vi "Auto Shooter Loop.vi"(4 "Right Shooter RPM":dbl, 6 "Left Shooter RPM":dbl, 10 "Vision Packet":T1, 11 "Shooter Presets":T2) -> ()   [LabVIEW 2016]
uses:
  Robot Global Data.vi
  Common Code/Auto Shoot Commands.ctl
  Common Code/Shooter Presets.ctl
  Common Code/Vision Packet.ctl
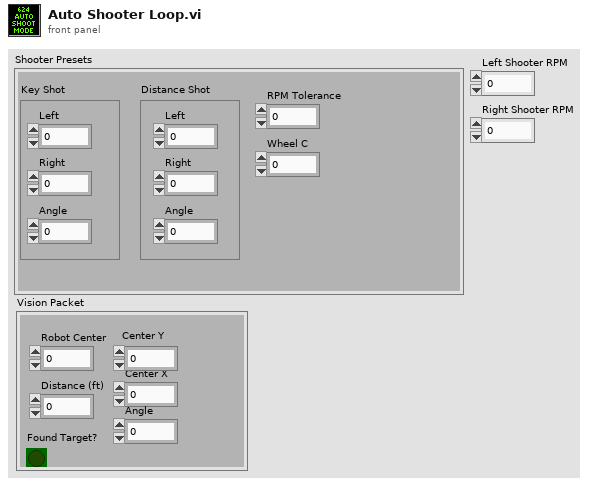
[diagram p1: front panel]
types:
  T1 = typedef "Vision Packet.ctl" = cluster{"Robot Center ":dbl, "Distance (ft)":dbl, "Center X":dbl, "Center Y":dbl, "Angle":dbl, "Found Target?":bool}
  T2 = typedef "Shooter Presets.ctl" = cluster{"Key Shot":cluster{"Left ":dbl, "Right":dbl, "Angle":dbl}, "Distance Shot":cluster{"Left":dbl, "Right":dbl, "Angle":dbl}, "RPM Tolerance":dbl, "Wheel C":dbl}
  T3 = typedef "Auto Shoot Commands.ctl" = enum16{"Idle", "Warmup", "Shoot"}
  T4 = typedef "Shooter Command Cluster.ctl" = cluster{"Y Power":dbl, "Modes":T5, "Shot Types":T6, "Auto Commands":T3}
  T5 = typedef "Shooter Modes.ctl" = enum16{"Manual", "Auto"}
  T6 = typedef "Shot Types.ctl" = enum16{"Key", "Distance"}
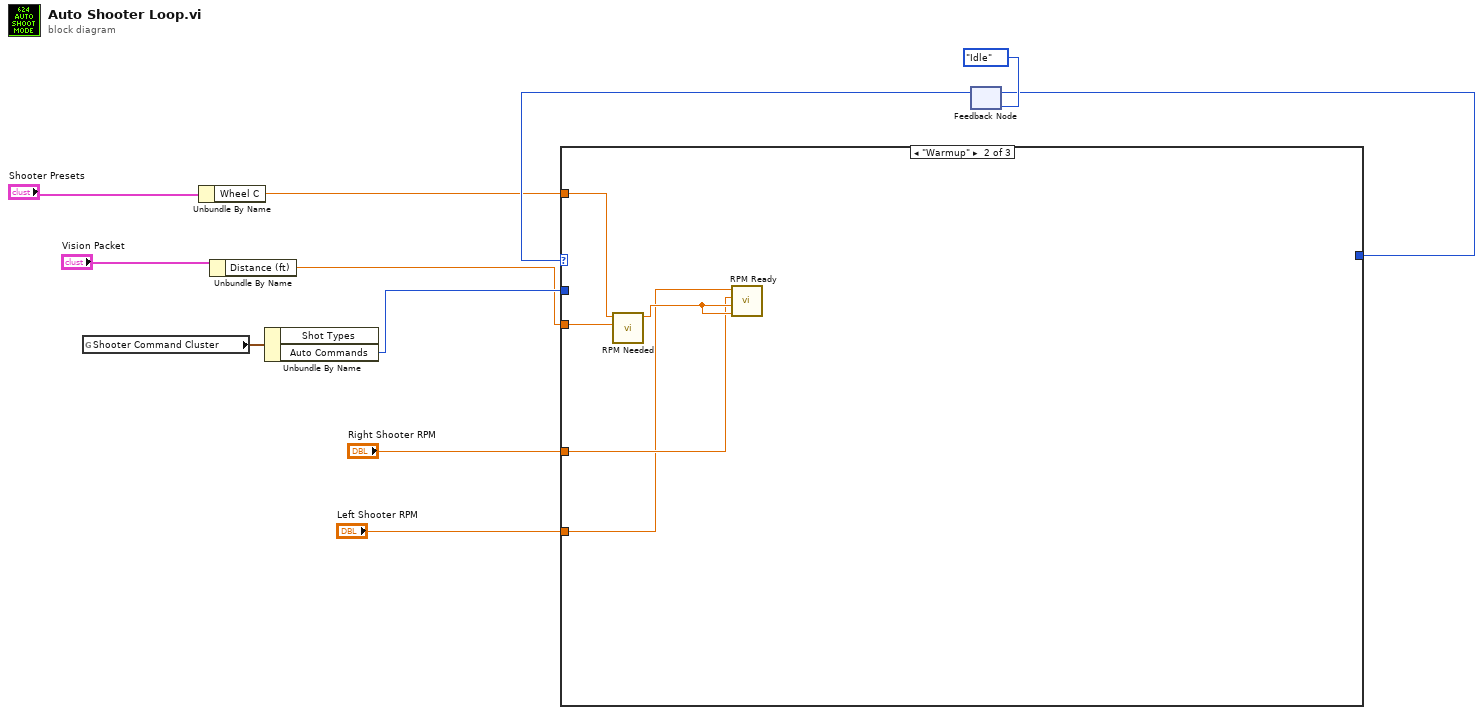
[diagram p0: block diagram]
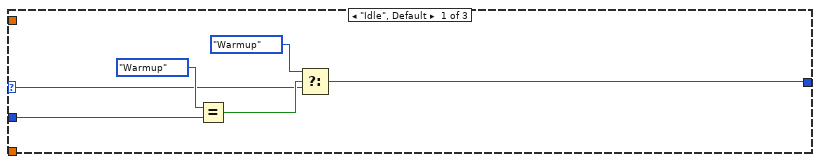
[diagram p2: hidden frame]
diagram:
  n1 = global read "Robot Global Data.vi" "Shooter Command Cluster"() -> (w11:T4)
  n2 = Unbundle By Name("Shooter Presets") -> ("Wheel C"=w4:dbl)
  n3 = Unbundle By Name("Vision Packet") -> ("Distance (ft)"=w3:dbl)
  n4 = Unbundle By Name(w11) -> ("Auto Commands"=w7:T3)  [unwired: 1 out]
  n5 = feedback #1(Auto_Shoot_Commands."Idle" ("Auto Commands")) -> (w8:T3)
  n6 = case shown="\"Warmup\"" w8 {
    selector: w8 -> [w12 _ _]
    tunnel: [w14 _ _] -> w9
    tunnel: w7 -> [w17 _ _]
    tunnel: w4 -> [_ w22 _]
    tunnel: w3 -> [_ w21 _]
    tunnel: "Right Shooter RPM" -> [_ w19 _]
    tunnel: "Left Shooter RPM" -> [_ w18 _]
    frame "Idle", Default {
      n7 = Equal?(x=Auto_Shoot_Commands."Warmup" ("Auto Commands"), y=w17) -> (x = y?=w15:bool)
      n8 = Select(t=Auto_Shoot_Commands."Warmup" ("Auto Commands"), s=w15, f=w12) -> (s? t:f=w14:T3)
    }
    frame "Warmup" {
      n9 = call "RPM Needed.vi"("Distance"=w21, "Wheel Circumference"=w22) -> ("RPM"=w20:dbl)  [unwired: 9 in]
      n10 = call "RPM Ready.vi"("Right RPM Target"=w20, "Left RPM Target"=w20, "Right RPM"=w19, "Left RPM"=w18) -> ()  [unwired: 7 in, 1 out]
    }
    frame "Shoot" {
    }
  }
  n11 = feedback-in #1(w9) -> ()
